vi "calculateHoldtime.vi"(9 "Current Time":dbl, 10 "Settling Time":dbl[unit], 11 "FirstTime":dbl) -> (2 "Delta":dbl, 3 "Boolean":bool)   [LabVIEW 2015]
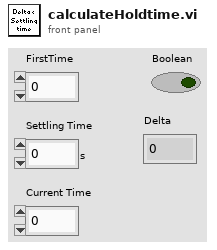
[diagram p1: front panel]
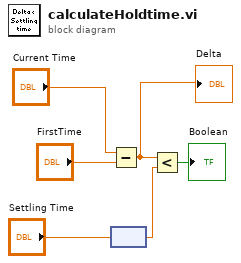
[diagram p0: block diagram]
diagram:
  n1 = Subtract(x="Current Time", y="FirstTime") -> (x-y=w1:dbl)
  "Delta" <- w1
  n2 = node("Settling Time") -> (w4:dbl)
  n3 = Less?(x=w1, y=w4) -> (x < y?=→"Boolean":bool)
